vi "ControlStatus.vi"(6 "state":T1, 7 "control refnum array in":refnum<vi>[](array[refnum]), 8 "error in (no error)":errorcluster) -> (0 "error out":errorcluster)   [LabVIEW 2009]
uses:
  Type Definitions/RCMControlStatus.ctl
  Support/Refnum/Private/FilteredControlRefnum (String Array)__slk_refnum.vi
  Support/Refnum/Library/Refnum.lvlib
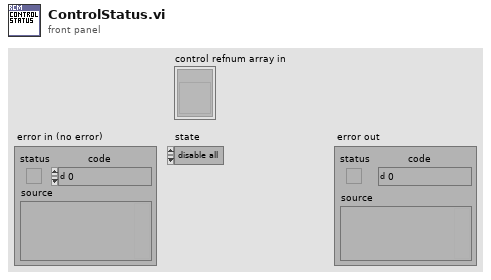
[diagram p1: front panel]
types:
  T1 = typedef "RCMControlStatus.ctl" = enum16{"disable all", "initialize", "enable save", "disable save", "enable tree edit", "disable tree edit", "enable item edit", "disable item edit", "user", "seperator"}
  T2 = enum8{"Enabled", "Disabled", "Disabled and Grayed Out"}
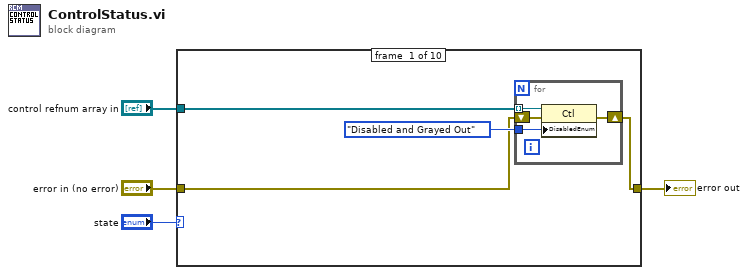
[diagram p0: block diagram]
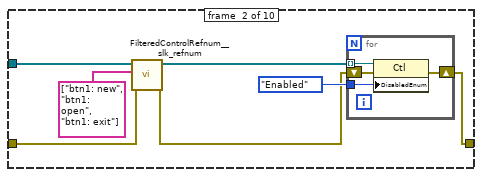
[diagram p2: hidden frame]
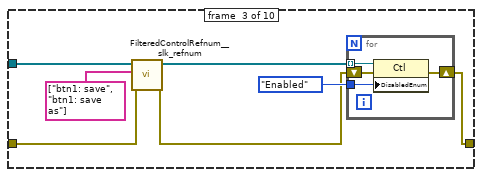
[diagram p3: hidden frame]
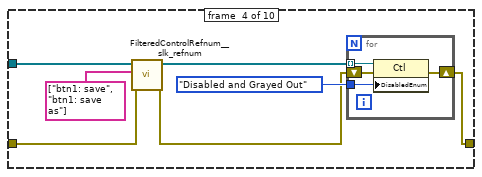
[diagram p4: hidden frame]
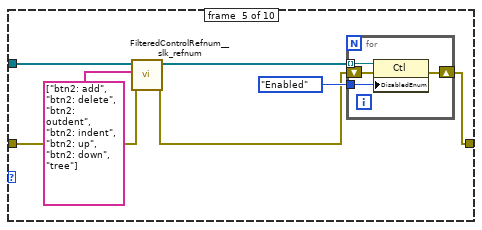
[diagram p5: hidden frame]
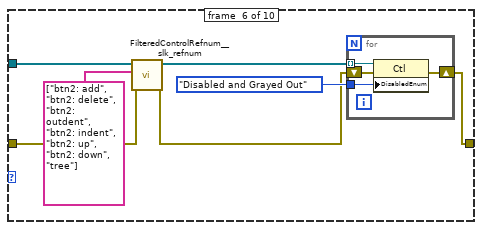
[diagram p6: hidden frame]
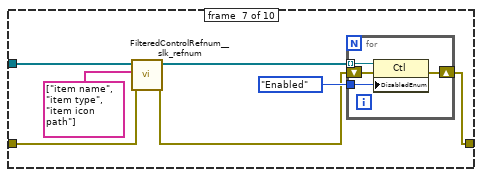
[diagram p7: hidden frame]
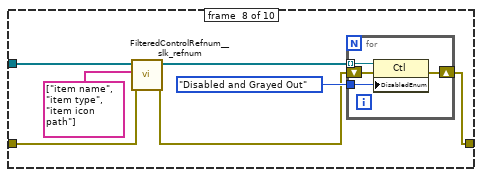
[diagram p8: hidden frame]
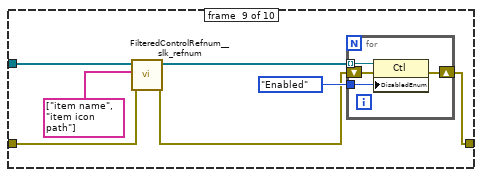
[diagram p9: hidden frame]
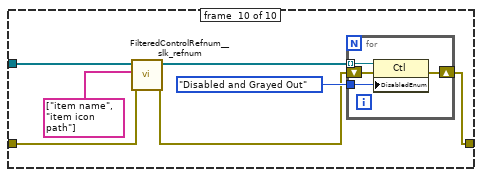
[diagram p10: hidden frame]
diagram:
  n1 = case shown="\"enable save\"" "state" {
    tunnel: "control refnum array in" -> [w8 w17 w28 w39 w50 w61 w72 w83 w94 w105]
    tunnel: "error in (no error)" -> [w6 w15 w26 w37 w48 w59 w70 w81 w92 w103]
    tunnel: [w5 w18 w29 w40 w51 w62 w73 w84 w95 w106] -> w1
    frame #0 {
      n2 = for {
        tunnel: w8 -> [w12] mode=indexing
        shift-right: [w11] -> w5
        shift-left: w6 -> [w10]
        tunnel: T2."Disabled and Grayed Out" ("Disabled") -> [w9]
        n3 = property class="Ctl"(reference=w12, error in=w10, "DisabledEnum"=w9) -> (error out=w11:errorcluster)  [unwired: 1 out]
      }
    }
    frame #1 {
      n4 = call-poly "FilteredControlRefnum__slk_refnum.vi"("error in (no error)"=w15, "filter"=string[] ["btn1: new", "btn1: open", "btn1: exit"], "control refnum array in"=w17) -> ("error out"=w14:errorcluster, "control refnum array out"=w16:refnum<vi>[])  [unwired: 6 in, 1 out]
      n5 = for {
        tunnel: w16 -> [w23] mode=indexing
        shift-right: [w22] -> w18
        shift-left: w14 -> [w21]
        tunnel: T2."Enabled" ("Disabled") -> [w20]
        n6 = property class="Ctl"(reference=w23, error in=w21, "DisabledEnum"=w20) -> (error out=w22:errorcluster)  [unwired: 1 out]
      }
    }
    frame #2 {
      n7 = call-poly "FilteredControlRefnum__slk_refnum.vi"("error in (no error)"=w26, "filter"=string[] ["btn1: save", "btn1: save as"], "control refnum array in"=w28) -> ("error out"=w25:errorcluster, "control refnum array out"=w27:refnum<vi>[])  [unwired: 6 in, 1 out]
      n8 = for {
        tunnel: w27 -> [w34] mode=indexing
        shift-right: [w33] -> w29
        shift-left: w25 -> [w32]
        tunnel: T2."Enabled" ("Disabled") -> [w31]
        n9 = property class="Ctl"(reference=w34, error in=w32, "DisabledEnum"=w31) -> (error out=w33:errorcluster)  [unwired: 1 out]
      }
    }
    frame #3 {
      n10 = call-poly "FilteredControlRefnum__slk_refnum.vi"("error in (no error)"=w37, "filter"=string[] ["btn1: save", "btn1: save as"], "control refnum array in"=w39) -> ("error out"=w36:errorcluster, "control refnum array out"=w38:refnum<vi>[])  [unwired: 6 in, 1 out]
      n11 = for {
        tunnel: w38 -> [w45] mode=indexing
        shift-right: [w44] -> w40
        shift-left: w36 -> [w43]
        tunnel: T2."Disabled and Grayed Out" ("Disabled") -> [w42]
        n12 = property class="Ctl"(reference=w45, error in=w43, "DisabledEnum"=w42) -> (error out=w44:errorcluster)  [unwired: 1 out]
      }
    }
    frame #4 {
      n13 = call-poly "FilteredControlRefnum__slk_refnum.vi"("error in (no error)"=w48, "filter"=string[] ["btn2: add", "btn2: delete", "btn2: outdent", "btn2: indent", "btn2: up", "btn2: down", "tree"], "control refnum array in"=w50) -> ("error out"=w47:errorcluster, "control refnum array out"=w49:refnum<vi>[])  [unwired: 6 in, 1 out]
      n14 = for {
        tunnel: w49 -> [w56] mode=indexing
        shift-right: [w55] -> w51
        shift-left: w47 -> [w54]
        tunnel: T2."Enabled" ("Disabled") -> [w53]
        n15 = property class="Ctl"(reference=w56, error in=w54, "DisabledEnum"=w53) -> (error out=w55:errorcluster)  [unwired: 1 out]
      }
    }
    frame #5 {
      n16 = call-poly "FilteredControlRefnum__slk_refnum.vi"("error in (no error)"=w59, "filter"=string[] ["btn2: add", "btn2: delete", "btn2: outdent", "btn2: indent", "btn2: up", "btn2: down", "tree"], "control refnum array in"=w61) -> ("error out"=w58:errorcluster, "control refnum array out"=w60:refnum<vi>[])  [unwired: 6 in, 1 out]
      n17 = for {
        tunnel: w60 -> [w67] mode=indexing
        shift-right: [w66] -> w62
        shift-left: w58 -> [w65]
        tunnel: T2."Disabled and Grayed Out" ("Disabled") -> [w64]
        n18 = property class="Ctl"(reference=w67, error in=w65, "DisabledEnum"=w64) -> (error out=w66:errorcluster)  [unwired: 1 out]
      }
    }
    frame #6 {
      n19 = call-poly "FilteredControlRefnum__slk_refnum.vi"("error in (no error)"=w70, "filter"=string[] ["item name", "item type", "item icon path"], "control refnum array in"=w72) -> ("error out"=w69:errorcluster, "control refnum array out"=w71:refnum<vi>[])  [unwired: 6 in, 1 out]
      n20 = for {
        tunnel: w71 -> [w78] mode=indexing
        shift-right: [w77] -> w73
        shift-left: w69 -> [w76]
        tunnel: T2."Enabled" ("Disabled") -> [w75]
        n21 = property class="Ctl"(reference=w78, error in=w76, "DisabledEnum"=w75) -> (error out=w77:errorcluster)  [unwired: 1 out]
      }
    }
    frame #7 {
      n22 = call-poly "FilteredControlRefnum__slk_refnum.vi"("error in (no error)"=w81, "filter"=string[] ["item name", "item type", "item icon path"], "control refnum array in"=w83) -> ("error out"=w80:errorcluster, "control refnum array out"=w82:refnum<vi>[])  [unwired: 6 in, 1 out]
      n23 = for {
        tunnel: w82 -> [w89] mode=indexing
        shift-right: [w88] -> w84
        shift-left: w80 -> [w87]
        tunnel: T2."Disabled and Grayed Out" ("Disabled") -> [w86]
        n24 = property class="Ctl"(reference=w89, error in=w87, "DisabledEnum"=w86) -> (error out=w88:errorcluster)  [unwired: 1 out]
      }
    }
    frame #8 {
      n25 = call-poly "FilteredControlRefnum__slk_refnum.vi"("error in (no error)"=w92, "filter"=string[] ["item name", "item icon path"], "control refnum array in"=w94) -> ("error out"=w91:errorcluster, "control refnum array out"=w93:refnum<vi>[])  [unwired: 6 in, 1 out]
      n26 = for {
        tunnel: w93 -> [w100] mode=indexing
        shift-right: [w99] -> w95
        shift-left: w91 -> [w98]
        tunnel: T2."Enabled" ("Disabled") -> [w97]
        n27 = property class="Ctl"(reference=w100, error in=w98, "DisabledEnum"=w97) -> (error out=w99:errorcluster)  [unwired: 1 out]
      }
    }
    frame #9 {
      n28 = call-poly "FilteredControlRefnum__slk_refnum.vi"("error in (no error)"=w103, "filter"=string[] ["item name", "item icon path"], "control refnum array in"=w105) -> ("error out"=w102:errorcluster, "control refnum array out"=w104:refnum<vi>[])  [unwired: 6 in, 1 out]
      n29 = for {
        tunnel: w104 -> [w111] mode=indexing
        shift-right: [w110] -> w106
        shift-left: w102 -> [w109]
        tunnel: T2."Disabled and Grayed Out" ("Disabled") -> [w108]
        n30 = property class="Ctl"(reference=w111, error in=w109, "DisabledEnum"=w108) -> (error out=w110:errorcluster)  [unwired: 1 out]
      }
    }
  }
  "error out" <- w1
